vi "Generate-ROI x-axis values array.vi"(4 "[ROI Time(us)]":dbl[](array[numeric]), 6 "Header data":T1={"Number of POI"=0, "Number of Miniscans"=0, "Number of Trials"=0, "Number of Cycles "=0, "# Averaged Frames"=0, "Laser power (%)"=0, "Pockels"=0.0, "Acquisition Length (sec)"=0.0, "Fill time (us)"=0.0, "DwellTime (us)"=0.0, "Miniscan Dwell time per pixel (us)"=0.0, "PMT 1"=0.0, "PMT 2"=0.0, "Back Apperture"=0.0, "Zoom"=0.0, "Number of Pixels in Miniscan"=0, "Frame Size"=200, "Field of View"=0.0, "X centre"=0.0, "Y centre"=0.0, "AOL Z"=0.0} {"Frame Size" items=["100X100"=100, "128X128"=128, "200X200"=200, "256X256"=256, "512X512"=512, "1024x1024"=1024, "2048x2048"=2048]; "Back Apperture" format="%#.6g"; "Pockels" format="%#.6g"; "PMT 2" format="%#.6g"; "PMT 1" format="%#.6g"; "Miniscan Dwell time per pixel (us)" format="%#.6g"; "Zoom" format="%#.6g"; "DwellTime (us)" format="%#.6g"; "Acquisition Length (sec)" format="%#.6g"; "Fill time (us)" format="%#.6g"}, 7 "Number of points in Y-axis array":i32, 9 "ROI number":i32, 10 "Type":T3, 11 "Pixels in ROI":i32) -> (2 "ROI X-axis values array (sec)":sgl[](array[numeric]))   [LabVIEW 2020]
uses:
  xcontrol/Interface VIs/Interface typedefs/Interface-ROI type enum.ctl
  Experiment header interface/Typedefs/Header parameters cluster-Zstack.ctl
  Typedefs/Frame Size.ctl
panel:
  # "Zstack header parameters"
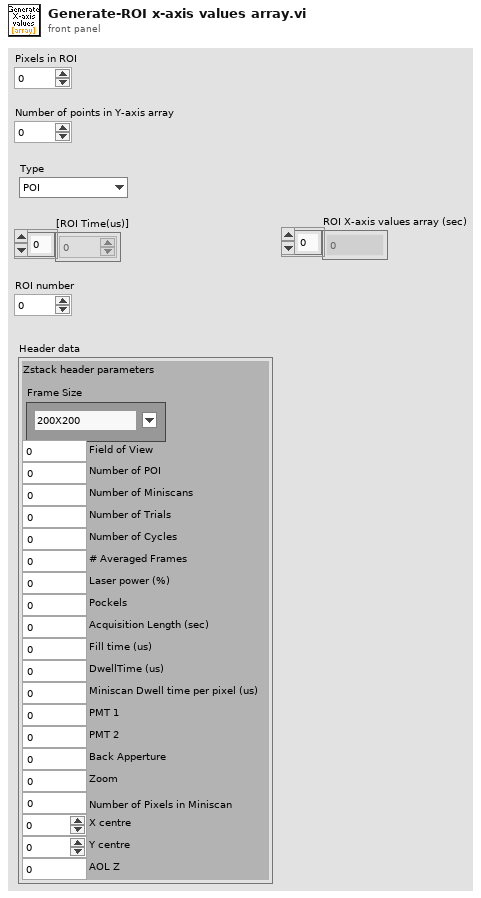
[diagram p1: front panel]
types:
  T1 = typedef "Header parameters cluster-Zstack.ctl" = cluster{"Number of POI":u16, "Number of Miniscans":u16, "Number of Trials":u16, "Number of Cycles ":u16, "# Averaged Frames":u16, "Laser power (%)":u8, "Pockels":dbl, "Acquisition Length (sec)":dbl, "Fill time (us)":dbl, "DwellTime (us)":dbl, "Miniscan Dwell time per pixel (us)":dbl, "PMT 1":dbl, "PMT 2":dbl, "Back Apperture":dbl, "Zoom":dbl, "Number of Pixels in Miniscan":u16, "Frame Size":T2, "Field of View":dbl, "X centre":dbl, "Y centre":dbl, "AOL Z":dbl}
  T2 = typedef "Frame Size.ctl" = u16
  T3 = typedef "Interface-ROI type enum.ctl" = enum16{"POI", "Mini-scan"}
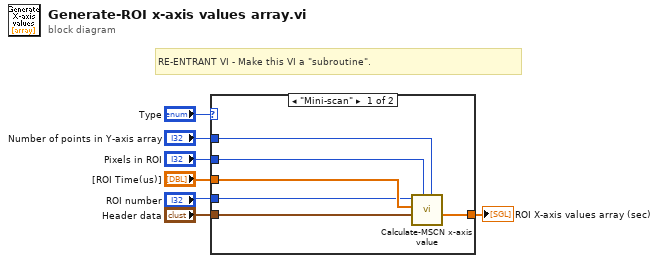
[diagram p0: block diagram]
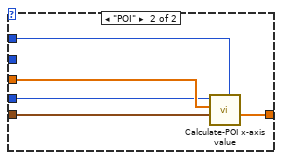
[diagram p2: hidden frame]
diagram:
  # "RE-ENTRANT VI - Make this VI a \"subroutine\"."
  n1 = case shown="\"Mini-scan\"" "Type" {
    tunnel: "Header data" -> [w13 w18]
    tunnel: "[ROI Time(us)]" -> [w12 w17]
    tunnel: "ROI number" -> [w11 w16]
    tunnel: "Pixels in ROI" -> [w10 _]
    tunnel: "Number of points in Y-axis array" -> [w9 w15]
    tunnel: [w8 w14] -> w7
    frame "Mini-scan" {
      n2 = call "Calculate-MSCN x-axis value.vi"("Total number of points in indexed ROI over the full experiment time"=w9, "Number of pixels in ROI"=w10, "Header Data"=w13, "[ROI Time(us)]"=w12, "ROI number"=w11) -> ("MSCN X-axis values array (sec)"=w8:sgl[])  [unwired: 6 in]
    }
    frame "POI" {
      n3 = call "Calculate-POI x-axis value.vi"("Total number of points in indexed ROI over the full experiment time"=w15, "Header Data"=w18, "[ROI Time(us)]"=w17, "ROI number"=w16) -> ("POI X-axis values array (sec)"=w14:sgl[])  [unwired: 7 in]
    }
  }
  "ROI X-axis values array (sec)" <- w7
